vi "APT_move_abs.vi"(1 "serial":i32=27004725, 2 "rel_pos":sgl) -> (0 "pfPosition":sgl)   [LabVIEW 2013]
panel:
  in  "Move\nAbs/ Rel":bool
  in  "abs_pos":sgl
  out "error out":errorcluster
  in  "MG17Motor":refnum<k7>(container)
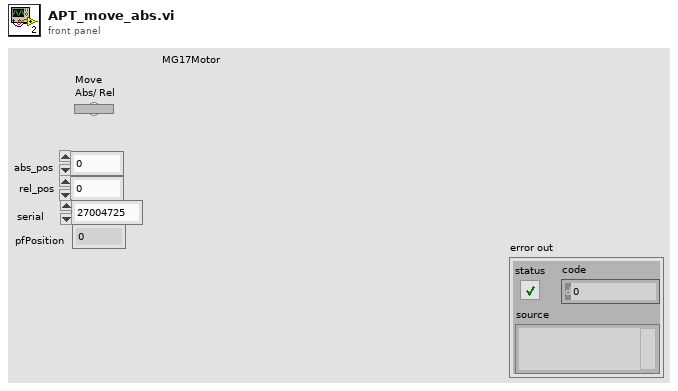
[diagram p1: front panel]
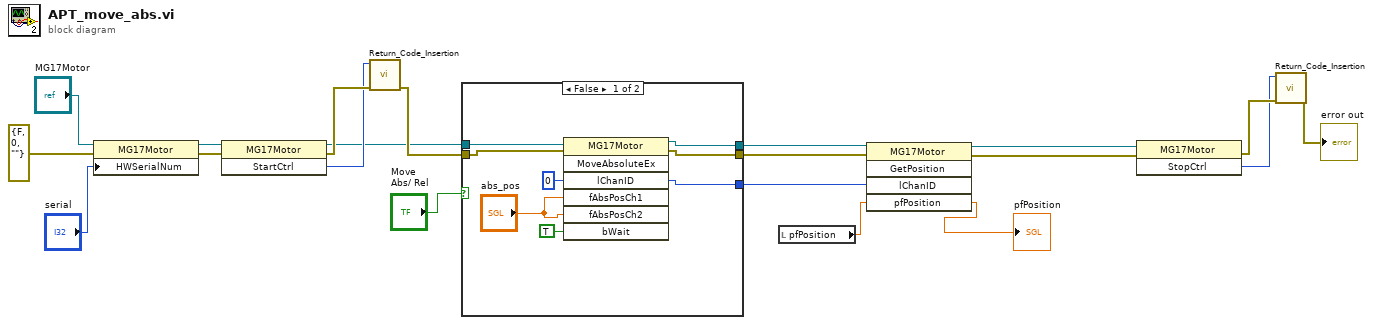
[diagram p0: block diagram]
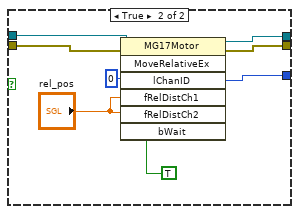
[diagram p2: hidden frame]
diagram:
  n1 = property class="MG17Motor"(reference="MG17Motor", error in=errorcluster {"status"=FALSE, "code"=0, "source"=""} ("error in (no error)"), "HWSerialNum"="serial") -> (reference out=w18:refnum<k7>, error out=w16:errorcluster)
  n2 = invoke class="MG17Motor" method="StartCtrl"(reference=w18, error in=w16) -> (reference out=w7:refnum<k7>, error out=w15:errorcluster, "StartCtrl"=w14:i32)  [unwired: 1 in]
  n3 = call "Return_Code_Insertion.vi"("error in (no error)"=w15, "Return Code"=w14) -> ("error out"=w8:errorcluster)  [unwired: 9 in]
  n4 = case shown="False" "Move\nAbs/ Rel" {
    tunnel: w8 -> [w27 w33]
    tunnel: w7 -> [w28 w32]
    tunnel: [w25 w31] -> w6
    tunnel: [w26 w30] -> w5
    tunnel: [w24 w29] -> w2
    frame False {
      n5 = invoke class="MG17Motor" method="MoveAbsoluteEx"(reference=w28, error in=w27, "lChanID"=0, "fAbsPosCh1"="abs_pos", "fAbsPosCh2"="abs_pos", "bWait"=TRUE) -> (reference out=w26:refnum<k7>, error out=w25:errorcluster, "lChanID"=w24:i32)  [unwired: 1 in, 4 out]
    }
    frame True {
      n6 = invoke class="MG17Motor" method="MoveRelativeEx"(reference=w32, error in=w33, "lChanID"=0, "fRelDistCh1"="rel_pos", "fRelDistCh2"="rel_pos", "bWait"=TRUE) -> (reference out=w30:refnum<k7>, error out=w31:errorcluster, "lChanID"=w29:i32)  [unwired: 1 in, 4 out]
    }
  }
  n7 = local read "pfPosition"() -> (w10:sgl)
  n8 = invoke class="MG17Motor" method="GetPosition"(reference=w5, error in=w6, "lChanID"=w2, "pfPosition"=w10) -> (reference out=w3:refnum<k7>, error out=w4:errorcluster, "pfPosition"=→"pfPosition":sgl)  [unwired: 1 in, 2 out]
  n9 = invoke class="MG17Motor" method="StopCtrl"(reference=w3, error in=w4) -> (error out=w13:errorcluster, "StopCtrl"=w12:i32)  [unwired: 1 in, 1 out]
  n10 = call "Return_Code_Insertion.vi"("error in (no error)"=w13, "Return Code"=w12) -> ("error out"=→"error out":errorcluster)  [unwired: 9 in]
